vi "Abort.vi"(8 "error in (no error)":errorcluster, 11 "AutomationContext in":refnum<class "AutomationContext.lvclass">) -> (0 "error out":errorcluster, 3 "AutomationContext out":refnum<class "AutomationContext.lvclass">)   [LabVIEW 2023, in "Automation.lvlib" / "AutomationContext.lvclass"]
uses:
  AutomationContext.lvclass
  AutomationContext.lvclass/AutomationContext.ctl
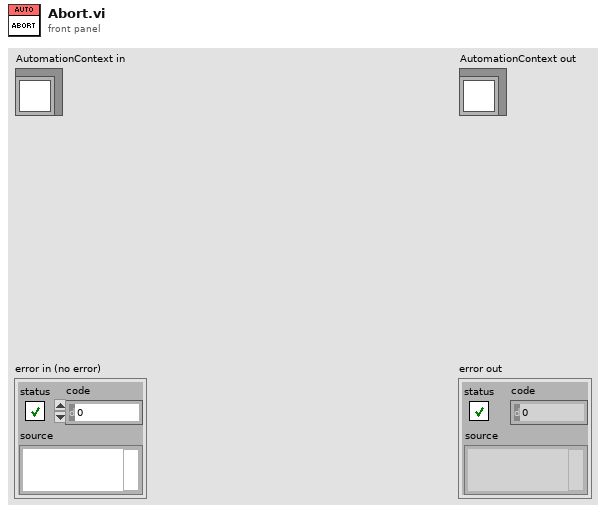
[diagram p1: front panel]
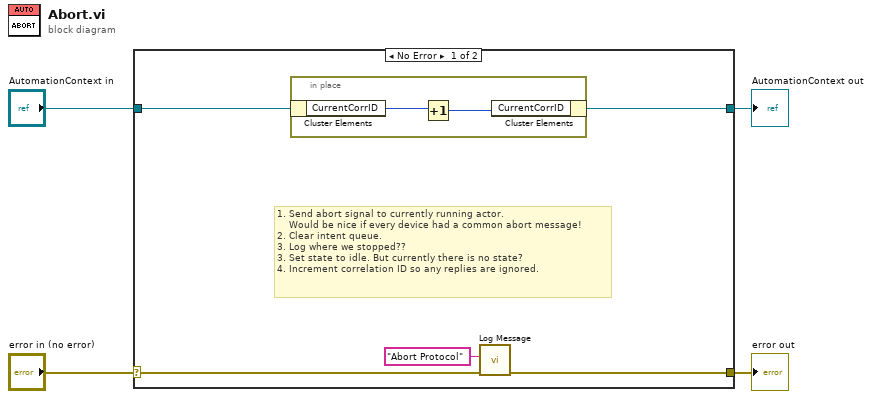
[diagram p0: block diagram]
diagram:
  n1 = case shown="No Error" "error in (no error)" {
    selector: "error in (no error)" -> [w9 w13]
    tunnel: [w8 w13] -> w3
    tunnel: [w5 w12] -> w1
    tunnel: "AutomationContext in" -> [w6 w12]
    frame No Error {
      # "1. Send abort signal to currently running actor.\n    Would be nice if every device had a common abort message!\n2. Clear intent queue.\n3. Log where we stopped??\n3. Set state to idle. But currently there is no state?\n4. Increment correlation ID so any replies are ignored."
      n2 = in-place {
        n3 = in-place-cluster #1(w6) -> ("CurrentCorrID"=w11:u32)
        n4 = Increment(x=w11) -> (x+1=w10:u32)
        n5 = in-place-cluster #1("CurrentCorrID"=w10) -> (w5:refnum<class "AutomationContext.lvclass">)
      }
      n6 = call "Log Message.vi"("error constant"=w9, "input"="Abort Protocol") -> ("error constant 2"=w8:errorcluster)  [unwired: 8 in, 1 out]
    }
    frame Error {
    }
  }
  "error out" <- w3
  "AutomationContext out" <- w1
